vi "Prepare.vi"(8 "error in (no error)":errorcluster, 10 "SQL":string, 11 "SQLite Connection in":refnum<class "Connection.lvclass">) -> (0 "error out":errorcluster, 1 "Rest of SQL":string, 2 "SQL Statement out":refnum<class "SQL Statement.lvclass">, 3 "SQLite Connection out":refnum<class "Connection.lvclass">, 4 "Valid Statement":bool)   [LabVIEW 2023, in "SQLite.lvlib" / "Connection.lvclass"]
doc: "Prepares (compiles) a single SQL statement for later execution. If the SQL contains parameters, then values can be \"bound\" to these parameters using a property node and the \"Bind\" properties. Prepares SQL statements are exectuted by calling \"First Step\". If data is returned it can be accessed using the \"Column\" properties, and multiple returned rows can be stepped through using \"Step\". After completion, the prepared statement can be \"Reset\" and reused, or it can be released (destroyed) using \"Finalize\"."
uses:
  Connection.lvclass
  SQLite.lvlib
  SQL Statement/SQL Statement.lvclass
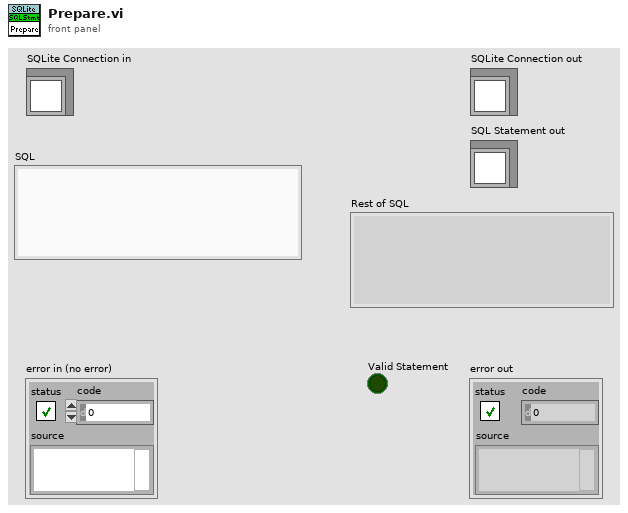
[diagram p1: front panel]
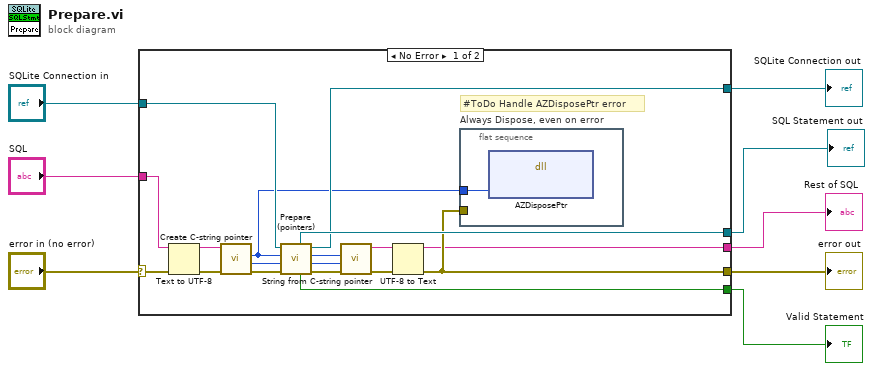
[diagram p0: block diagram]
diagram:
  n1 = case shown="No Error" "error in (no error)" {
    selector: "error in (no error)" -> [w25 w29]
    tunnel: [w23 w29] -> w7
    tunnel: [w21 w28] -> w5
    tunnel: "SQLite Connection in" -> [w22 w28]
    tunnel: "SQL" -> [w26 _]
    tunnel: [w24 _] -> w3
    tunnel: [w20 _] -> w2
    tunnel: [w19 _] -> w1
    frame No Error {
      # "#ToDo Handle AZDisposePtr error"
      n2 = Text to UTF-8(8:w25, 11:w26) -> (0:w17:errorcluster, 3:w18:string)  [unwired: 1 in]
      n3 = call "Create C-string pointer.vi"("error in (no error)"=w17, "string"=w18) -> ("error out"=w14:errorcluster, "size"=w16:i32, "C-string pointer"=w11:i64)  [unwired: 6 in, 1 out]
      n4 = call "Prepare (pointers).vi"("error in (no error)"=w14, "Bytes in SQL"=w16, "SQL pointer"=w11, "SQLite Connection in"=w22) -> ("error out"=w13:errorcluster, "Remaining bytes"=w12:i32, "Remaining SQL Tail"=w15:i64, "SQLite Connection out"=w21:refnum<class "Connection.lvclass">, "Valid Statement"=w19:bool, "SQL Statement out"=w24:refnum<class "SQL Statement.lvclass">)  [unwired: 2 in]
      n5 = call "String from C-string pointer.vi"("error in (no error)"=w13, "Bytes to copy"=w12, "Pointer"=w15) -> ("error out"=w10:errorcluster, "string"=w9:string)  [unwired: 7 in]
      n6 = UTF-8 to Text(8:w10, 11:w9) -> (0:w23:errorcluster, 3:w20:string)  [unwired: 1 in]
      n7 = flat-sequence "Always Dispose, even on error" {
        tunnel: w11 -> [w27]
        tunnel: w23 -> [_]
        frame #0 {
          n8 = dll-call lib="LabVIEW" fn="AZDisposePtr"("pointer"=w27) -> ()  [unwired: 5 in, 2 out]
        }
      }
    }
    frame Error {
    }
  }
  "error out" <- w7
  "SQLite Connection out" <- w5
  "SQL Statement out" <- w3
  "Rest of SQL" <- w2
  "Valid Statement" <- w1
